vi "read config.vi"(8 "error in (no error)":errorcluster, 10 "Path":path, 11 "USB IO in":refnum<class "USB IO.lvclass">) -> (0 "error out":errorcluster, 3 "USB IO out":refnum<class "USB IO.lvclass">)   [LabVIEW 2025, in "USB IO.lvlib" / "USB IO.lvclass"]
uses:
  USB IO.lvclass
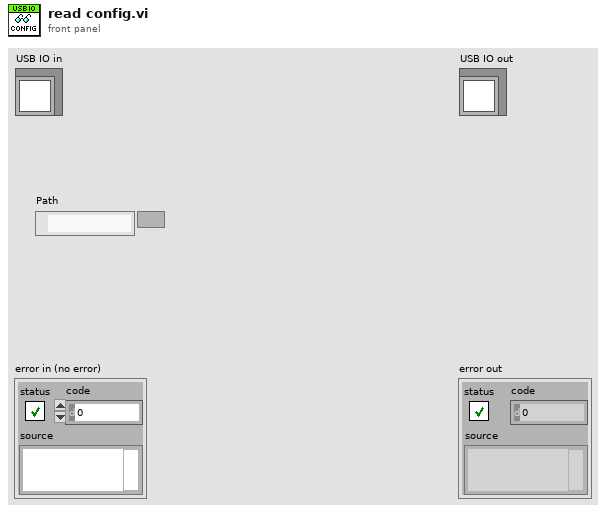
[diagram p1: front panel]
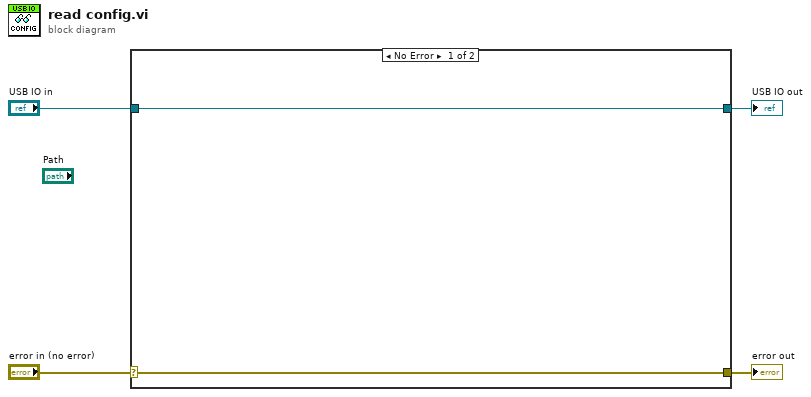
[diagram p0: block diagram]
diagram:
  n1 = case shown="No Error" "error in (no error)" {
    selector: "error in (no error)" -> [w5 w8]
    tunnel: [w5 w8] -> w3
    tunnel: [w6 w7] -> w1
    tunnel: "USB IO in" -> [w6 w7]
    frame No Error {
    }
    frame Error {
    }
  }
  "error out" <- w3
  "USB IO out" <- w1
